vi "RegisterUIMessage.vi"(8 "error in (no error)":errorcluster, 9 "UIMsg":refnum<class "SendMessage.lvclass">, 11 "VXMx2 in":refnum<class "VXMx2.lvclass">) -> (0 "error out":errorcluster, 3 "VXMx2 out":refnum<class "VXMx2.lvclass">)   [LabVIEW 2018, in "VXMx2.lvclass"]
doc: "Copy in a live UI message object so that it can be used from inside the VXM controller object."
uses:
  VXMx2.lvclass
  SendMessage/SendMessage.lvclass
  VXMx2.lvclass/VXMx2.ctl
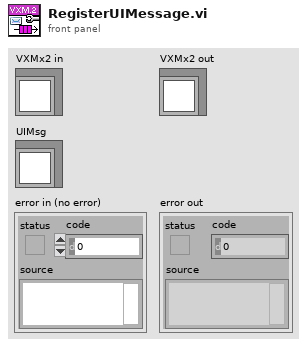
[diagram p1: front panel]
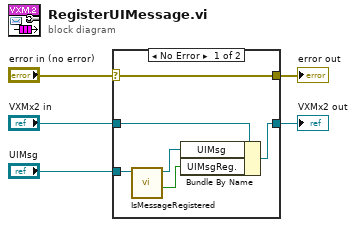
[diagram p0: block diagram]
diagram:
  n1 = case shown="No Error" "error in (no error)" {
    selector: "error in (no error)" -> [w10 w13]
    tunnel: [w10 w13] -> w4
    tunnel: [w9 w12] -> w2
    tunnel: "VXMx2 in" -> [w11 w12]
    tunnel: "UIMsg" -> [w8 _]
    frame No Error {
      n2 = call "IsMessageRegistered.vi"("SendMessage in"=w8) -> ("Message Que is Registered"=w6:bool, "SendMessage out"=w7:refnum<class "SendMessage.lvclass">)  [unwired: 8 in, 1 out]
      n3 = Bundle By Name(cluster=w11, "UIMsg"=w7, "UIMsgReg."=w6) -> (w9:refnum<class "VXMx2.lvclass">)
    }
    frame Error {
    }
  }
  "error out" <- w4
  "VXMx2 out" <- w2
